vi "PicoScope4000aExampleStreaming.vi"(1 "stop":bool, 5 "Open Using Serial Number":bool, 7 "Serial Number":string) -> ()   [LabVIEW 2010]
doc: "This example demonstrates how to use the PicoScope Labview library to stream data from a PicoScope 5000 Series Device"
uses:
  PicoScope4000aLib/PicoScope4000aAnalogChannelSettings.ctl
  shared/Buffer and Transfer Settings.ctl
panel:
  in  "Write to TDMS":bool
  out "Unit Info":T1
  in  "Trigger Settings":T2={"Trigger Enabled"=FALSE, "Trigger Source"=enum."Channel A", "Trigger Threshold (Volts/Probe units)"=0.0, "Trigger Direction"=2, "Trigger Delay (samples)"=0, "Auto Trigger Time (ms)"=1000} {"Trigger Direction" items=["Rising"=2, "Falling"=3]}
  out "Analog Channels":cluster{i32, dbl, "Data (Volts)":dbl[]}[](graph)
  in  "Channel B Settings":T3={"Enabled"=TRUE, "Coupling"=1, "Range"=6, "Analogue Offset"=0.0, "Bandwidth Limit"=0} {"Bandwidth Limit" items=["Full", "20kHz", "100kHz", "1MHz"]; "Range" items=["10 mV", "20 mV", "50 mV", "100 mV", "200 mV", "500 mV", "1 V", "2 V", "5 V", "10 V", "20 V", "50 V ", "100 V"]; "Coupling" items=["AC", "DC"]}
  in  "Channel A Settings":T3={"Enabled"=TRUE, "Coupling"=1, "Range"=6, "Analogue Offset"=0.0, "Bandwidth Limit"=0} {"Bandwidth Limit" items=["Full", "20kHz", "100kHz", "1MHz"]; "Range" items=["10 mV", "20 mV", "50 mV", "100 mV", "200 mV", "500 mV", "1 V", "2 V", "5 V", "10 V", "20 V", "50 V ", "100 V"]; "Coupling" items=["AC", "DC"]}
  out "Raw Sample Interval (sec)":dbl format="%#.5p"
  out "Max ADC value":i16
  out "Chunk time(ms)":u32
  out "Elapsed time":dbl
  in  "Data file":path=path "PicoScope4000aExampleStreaming Data"
  out "Queue depth":i32(graph)
  out "queue depth":i32
  in  "Buffer and Transfer Settings":T4={"startIndex"=0, "Samples"=1000000, "Down Sample Ratio"=1, "Down-Sample Mode"=0} {"Down-Sample Mode" items=["RAW none"=2147483648, "None"=0, "Aggregate"=1, "Decimate"=2, "Average"=4]; "Down Sample Ratio" step=1; "Samples" format="%_6p"}
  out "USB Powered":bool
  out "USB 3.0 device on non-USB 3.0 Port":bool=TRUE
  out "TriggeredAt (In Buffer)":u32 format="%#.6p"
  out "TriggeredAt (Total samples)":u32 format="%#.6p"
  in  "Acquisition Settings":T5={"Auto Stop"=FALSE, "Desired Sample Interval"=100, "Pre-trigger Samples"=0, "Post-trigger Samples"=1000000, "Down-Sample Ratio"=1, "Down-Sample Mode"=0, "Time Units"=2} {"Time Units" items=["Nanoseconds (ns)"=2, "Microseconds (us)"=3, "Milliseconds (ms)"=4, "Seconds (s)"=5]; "Down-Sample Mode" items=["None"=0, "Aggregate"=1, "Decimate"=2, "Average"=4]; "Post-trigger Samples" format="%#.6p"; "Pre-trigger Samples" format="%#_6p"}
  out "Triggered":bool
  out "DownSample Interval (sec)":dbl format="%#.5p"
  out "Total Samples":u32 format="%#.6p"
  out "Auto Stopped":bool
  out "Number of Samples per Capture":u32 format="%#.6p"
  in  "Resolution":u32(ring)=1 items=["8-bit", "12-bit", "14-bit", "15-bit (max. 2 ch.)", "16-bit (max. 1 ch.)"]
  in  "Apply  Settings":bool
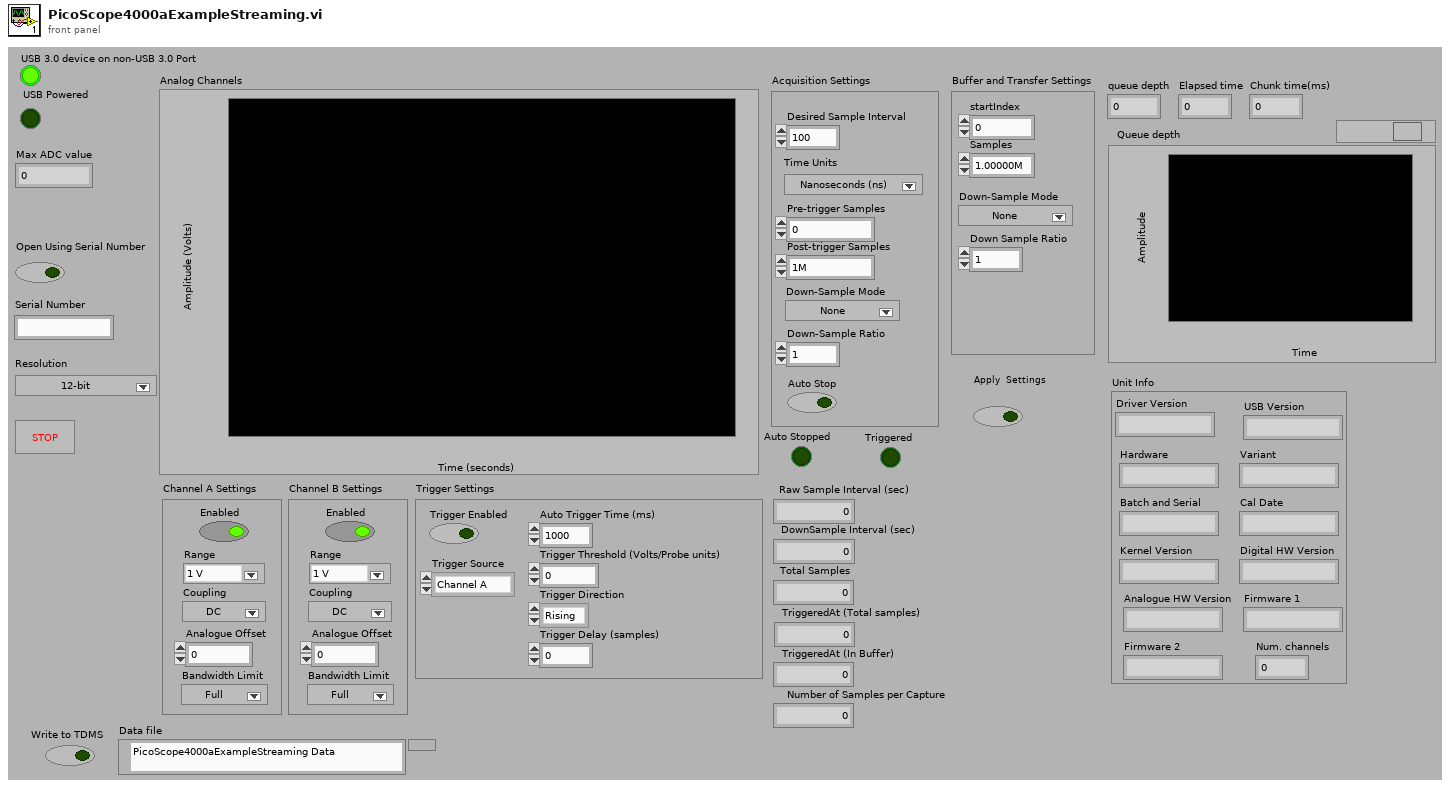
[diagram p1: front panel]
types:
  T1 = cluster{"Driver Version":string, "USB Version":string, "Hardware":string, "Variant":string, "Batch and Serial":string, "Cal Date":string, "Kernel Version":string, "Digital HW Version":string, "Analogue HW Version":string, "Firmware 1":string, "Firmware 2":string, "Num. channels":i16}
  T2 = cluster{"Trigger Enabled":bool, "Trigger Source":enum16{"Channel A", "Channel B", "Channel C", "Channel D", "Channel E", "Channel F", "Channel G", "Channel H"}, "Trigger Threshold (Volts/Probe units)":dbl, "Trigger Direction":u16, "Trigger Delay (samples)":u32, "Auto Trigger Time (ms)":i16}
  T3 = typedef "PicoScope4000aAnalogChannelSettings.ctl" = cluster{"Enabled":bool, "Coupling":i16, "Range":u32, "Analogue Offset":sgl, "Bandwidth Limit":u32}
  T4 = typedef "Buffer and Transfer Settings.ctl" = cluster{"startIndex":u64, "Samples":u64, "Down Sample Ratio":u64, "Down-Sample Mode":u32}
  T5 = cluster{"Auto Stop":bool, "Desired Sample Interval":u32, "Pre-trigger Samples":u32, "Post-trigger Samples":u32, "Down-Sample Ratio":u32, "Down-Sample Mode":i32, "Time Units":u32}
  T6 = enum16{"open", "open or create", "create or replace", "create", "open (read-only)"}
  T7 = cluster{"Channel A Buffer":i16[], "Channel B Buffer":i16[], "Channel C Buffer":i16[], "Channel D Buffer":i16[], "Channel E Buffer":i16[], "Channel F Buffer":i16[], "Channel G Buffer":i16[], "Channel H Buffer":i16[], "Port 0":i16[], "Port 1":i16[]}
  T8 = cluster{i32, "DownSample Interval (sec)":dbl, "Data":dbl[]}
  T9 = cluster{i32, "DownSample Interval (sec)":dbl, "Data":dbl[]}[]
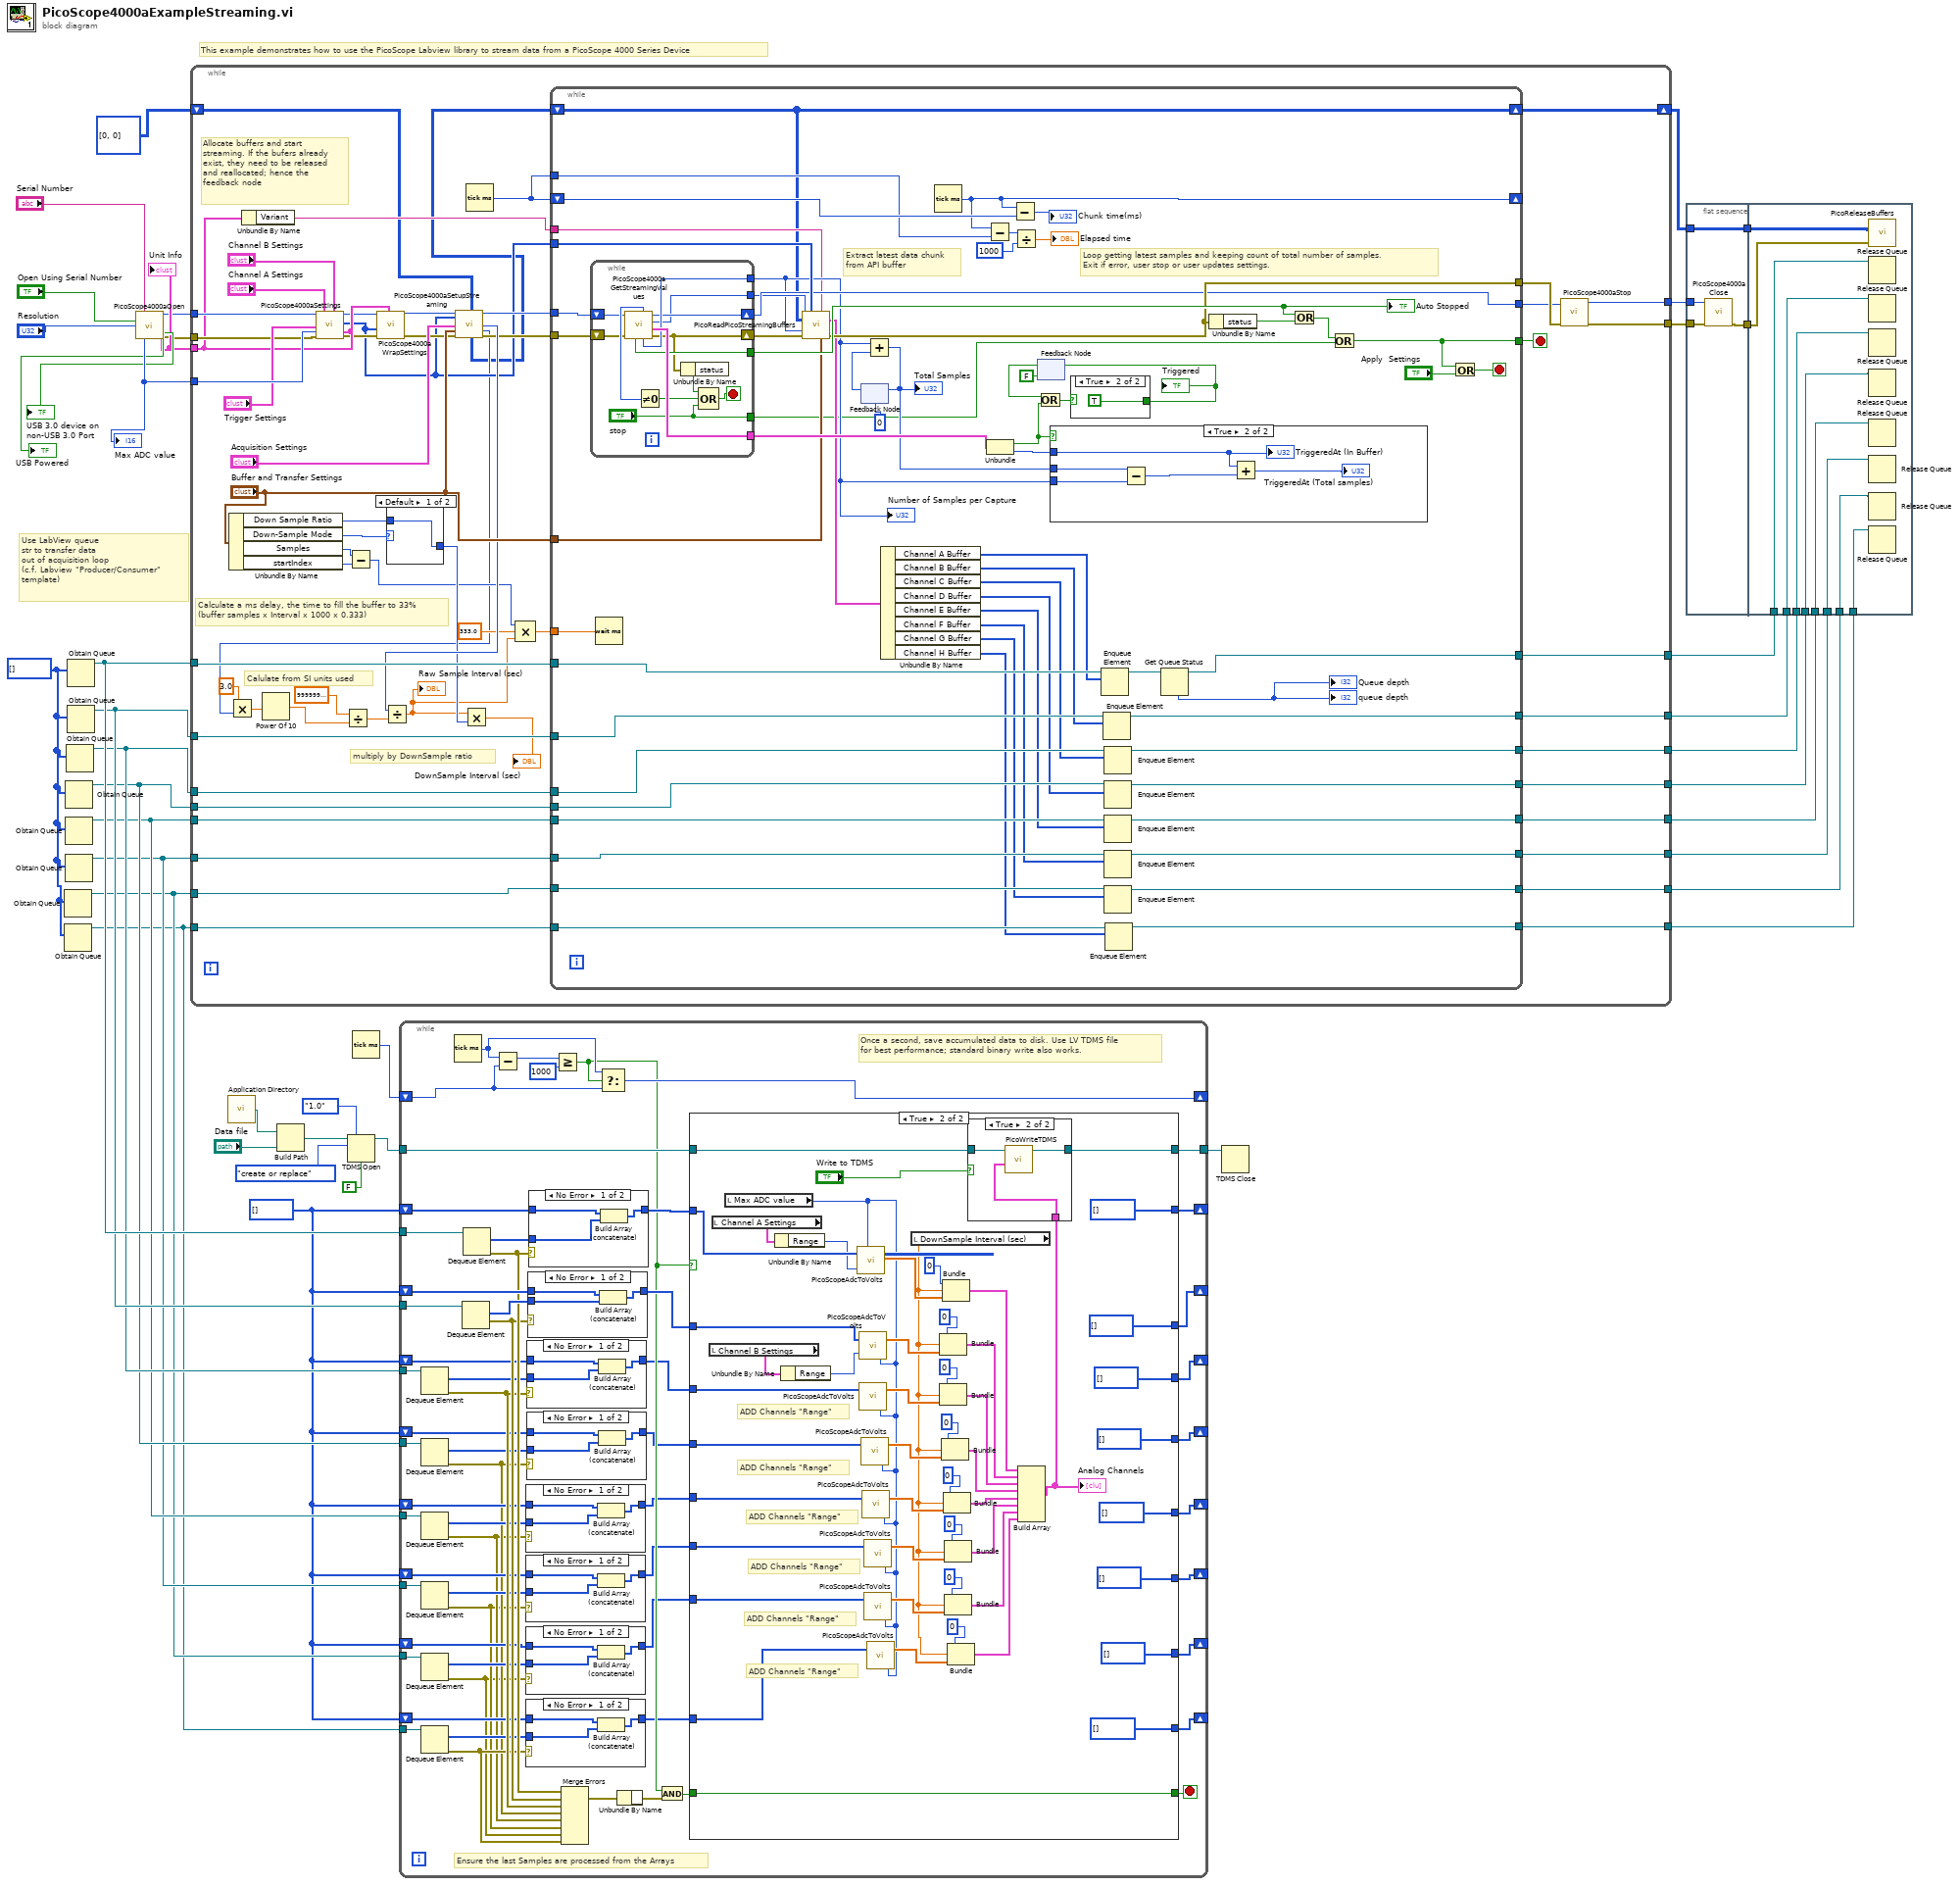
[diagram p0: block diagram]
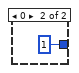
[diagram p12: hidden frame]
diagram:
  w8 = i16[] [] ("History Data")
  w21 = i16[] [] ("History Data")
  # "Use LabView queue\nstr to transfer data\nout of acquisition loop\n(c.f. Labview \"Producer/Consumer\"\ntemplate)"
  # "This example demonstrates how to use the PicoScope Labview library to stream data from a PicoScope 4000 Series Device"
  n1 = Obtain Queue(element data type=w21) -> (queue out=w10:refnum<queue>)  [unwired: 4 in, 2 out]
  n2 = Obtain Queue(element data type=w21) -> (queue out=w9:refnum<queue>)  [unwired: 4 in, 2 out]
  n3 = Obtain Queue(element data type=w21) -> (queue out=w13:refnum<queue>)  [unwired: 4 in, 2 out]
  n4 = Obtain Queue(element data type=w21) -> (queue out=w12:refnum<queue>)  [unwired: 4 in, 2 out]
  n5 = Obtain Queue(element data type=w21) -> (queue out=w11:refnum<queue>)  [unwired: 4 in, 2 out]
  n6 = Obtain Queue(element data type=w21) -> (queue out=w14:refnum<queue>)  [unwired: 4 in, 2 out]
  n7 = Obtain Queue(element data type=w21) -> (queue out=w38:refnum<queue>)  [unwired: 4 in, 2 out]
  n8 = Obtain Queue(element data type=w21) -> (queue out=w26:refnum<queue>)  [unwired: 4 in, 2 out]
  n9 = call "PicoScope4000aOpen.vi"("Serial Number"="Serial Number", "Use Serial Number"="Open Using Serial Number", "Resolution"="Resolution") -> ("handle"=w6:i16, "Unit Info"=w22:T1, "Max ADC value"=w39:i16, "USB powered"=→"USB 3.0 device on non-USB 3.0 Port":bool, "USB 3.0 on non-USB 3.0 port"=→"USB Powered":bool, "error out"=w5:errorcluster)  [unwired: 5 in, 2 out]
  "Max ADC value" <- w39
  "Unit Info" <- w22
  n10 = while {
    tunnel: [w87] -> w37
    tunnel: w22 -> [w54]
    tunnel: w39 -> [w100]
    tunnel: [w95] -> w36
    tunnel: w38 -> [w94]
    tunnel: [w93] -> w27
    tunnel: w26 -> [w92]
    tunnel: w14 -> [w74]
    tunnel: w13 -> [w73]
    tunnel: w12 -> [w72]
    tunnel: w11 -> [w71]
    tunnel: w10 -> [w70]
    tunnel: w9 -> [w69]
    tunnel: [w68] -> w20
    tunnel: [w67] -> w19
    tunnel: [w66] -> w18
    tunnel: [w65] -> w17
    tunnel: [w64] -> w16
    tunnel: [w63] -> w15
    tunnel: [w58] -> w7
    tunnel: w6 -> [w56]
    tunnel: w5 -> [w55]
    shift-right: [w43] -> w3
    shift-left: u64[][] [[0], [0]] ("Pointer array") -> [w45]
    stop <- w101 stop-if-true
    # "Calculate a ms delay, the time to fill the buffer to 33%\n(buffer samples x Interval x 1000 x 0.333)"
    # "multiply by DownSample ratio"
    # "Calulate from SI units used"
    # "Allocate buffers and start\nstreaming. If the bufers already\nexist, they need to be released\nand reallocated; hence the\nfeedback node"
    n11 = Unbundle By Name("Buffer and Transfer Settings") -> ("Down Sample Ratio"=w98:u64, "Down-Sample Mode"=w99:u32, "Samples"=w77:u64, "startIndex"=w76:u64)
    n12 = Unbundle By Name(w54) -> ("Variant"=w59:string)
    n13 = call "PicoScope4000aSettings.vi"("handle in"=w56, "Trigger Settings"="Trigger Settings", "Max ADC value"=w100, "error in"=w55, "Channel A Settings"="Channel A Settings", "Channel B Settings"="Channel B Settings", "Unit Info"=w54) -> ("handle out"=w52:i16, "Enabled array"=w47:i16[], "error out"=w53:errorcluster)  [unwired: 10 in]
    n14 = Subtract(x=w77, y=w76) -> (x-y=w61:u64)
    n15 = call "PicoScope4000aWrapSettings.vi"("Unit Info"=w54, "error in (no error)"=w53, "Enabled array"=w47, "Handle In"=w52) -> ("error out"=w49:errorcluster, "Handle Out"=w48:i16)  [unwired: 6 in]
    n16 = case shown="Default" w99 {
      tunnel: [w102 u32 1 ("Down-Sample Ratio")] -> w79
      tunnel: w98 -> [w102 _]
      frame Default {
      }
      frame 0 {
      }
    }
    n17 = call "PicoScope4000aSetupStreaming.vi"("handle in"=w48, "enabled array"=w47, "Acquisition Settings"="Acquisition Settings", "Buffer and Transfer Settings"="Buffer and Transfer Settings", "error in"=w49, "Pointers In"=w45) -> ("Pointer array"=w44:u64[][], "handle out"=w51:i16, "Sample Interval"=w80:u32, "sampleIntervalTimeUnits"=w46:u32, "error out"=w50:errorcluster)  [unwired: 9 in]
    n18 = Multiply(x=3.0, y=w46) -> (x*y=w85:dbl)
    n19 = Power Of 10(x=w85) -> (10^x=w84:dbl)
    n20 = Divide(x=sgl 1000000000000000.0 ("y"), y=w84) -> (x/y=w81:dbl)
    n21 = Divide(x=w80, y=w81) -> (x/y=w60:dbl)
    "Raw Sample Interval (sec)" <- w60
    n22 = Multiply(x=w60, y=w79) -> (x*y=→"DownSample Interval (sec)":dbl)
    n23 = Tick Count (ms)() -> (millisecond timer value=w86:u32)
    n24 = Compound Arithmetic op=MULTIPLY(w61, 333.0 ("value"), w60) -> (w78:dbl)
    n25 = while {
      tunnel: [w133] -> w88
      tunnel: [w165] -> w101
      tunnel: w51 -> [w150]
      tunnel: w50 -> [w149]
      tunnel: [w146] -> w89
      tunnel: "Buffer and Transfer Settings" -> [w148]
      tunnel: w47 -> [w145]
      tunnel: [w143] -> w95
      tunnel: w94 -> [w141]
      shift-right: [w135] -> _
      shift-left: w86 -> [w136]
      tunnel: w59 -> [w129]
      tunnel: [w124] -> w93
      tunnel: w92 -> [w128]
      tunnel: w86 -> [w125]
      tunnel: w78 -> [w105]
      tunnel: w74 -> [w123]
      tunnel: w73 -> [w122]
      tunnel: w72 -> [w121]
      tunnel: w71 -> [w120]
      tunnel: w70 -> [w119]
      tunnel: w69 -> [w118]
      tunnel: [w117] -> w68
      tunnel: [w116] -> w67
      tunnel: [w115] -> w66
      tunnel: [w114] -> w65
      tunnel: [w113] -> w64
      tunnel: [w112] -> w63
      shift-right: [w104] -> w43
      shift-left: w44 -> [w104]
      stop <- w164 stop-if-true
      # "Loop getting latest samples and keeping count of total number of samples. \nExit if error, user stop or user updates settings."
      # "Extract latest data chunk\nfrom API buffer"
      n26 = while {
        tunnel: [w179] -> w163
        tunnel: [w178] -> w160
        tunnel: [w167] -> w131
        tunnel: [w177] -> w130
        shift-right: [w168] -> w133
        shift-left: w150 -> [w171]
        shift-right: [w169] -> w147
        shift-left: w149 -> [w170]
        tunnel: ["stop"] -> w126
        stop <- w173 stop-if-true
        n27 = call "PicoScope4000aGetStreamingValues.vi"("error in"=w170, "handle in"=w171) -> ("error out"=w169:errorcluster, "Trigger"=w179:cluster{bool, "triggeredAt (Total samples)":u32}, "Start Index in Driver Buffer"=w167:u32, "handle out"=w168:i16, "Number of Samples"=w177:u32, "ready"=w176:i16, "Auto Stopped"=w178:bool)  [unwired: 3 in]
        n28 = Not Equal To 0?(x=w176) -> (x != 0?=w174:bool)
        n29 = Unbundle By Name(w169) -> ("status"=w175:bool)
        n30 = Compound Arithmetic op=OR(w175, w174, "stop") -> (w173:bool)
      }
      "Number of Samples per Capture" <- w130
      "Auto Stopped" <- w160
      n31 = Wait (ms)(milliseconds to wait=w105) -> ()  [unwired: 1 out]
      n32 = call "PicoReadPicoStreamingBuffers.vi"("enabled array"=w145, "Buffer and Transfer Settings"=w148, "Variant"=w129, "Pointer array"=w104, "Offset Index"=w131, "Number of Samples"=w130, "error in (no error)"=w147) -> ("Buffers (Max or non-aggregated)"=w140:T7, "error out"=w146:errorcluster)  [unwired: 6 in, 1 out]
      n33 = feedback #1(u32 0) -> (w156:u32)
      n34 = Add(x=w130, y=w156) -> (x+y=w154:u32)
      "Total Samples" <- w154
      n35 = feedback-in #1(w154) -> ()
      n36 = Unbundle By Name(w140) -> ("Channel A Buffer"=w132:i16[], "Channel B Buffer"=w127:i16[], "Channel C Buffer"=w111:i16[], "Channel D Buffer"=w110:i16[], "Channel E Buffer"=w109:i16[], "Channel F Buffer"=w108:i16[], "Channel G Buffer"=w107:i16[], "Channel H Buffer"=w106:i16[])
      n37 = Tick Count (ms)() -> (millisecond timer value=w135:u32)
      n38 = Subtract(x=w135, y=w125) -> (x-y=w139:u32)
      n39 = Unbundle(w163) -> (w152:bool, "triggeredAt (Total samples)"=w151:u32)
      n40 = Subtract(x=w135, y=w136) -> (x-y=→"Chunk time(ms)":u32)
      n41 = Divide(x=w139, y=u32 1000) -> (x/y=→"Elapsed time":dbl)
      n42 = feedback #2(FALSE) -> (w158:bool)
      n43 = Or(x=w158, y=w152) -> (x .or. y?=w155:bool)
      n44 = case shown="True" w152 {
        tunnel: w130 -> [_ w180]
        tunnel: w154 -> [_ w184]
        tunnel: w151 -> [_ w182]
        frame False {
        }
        frame True {
          n45 = Subtract(x=w184, y=w180) -> (x-y=w183:u32)
          n46 = Add(x=w182, y=w183) -> (x+y=→"TriggeredAt (Total samples)":u32)
          "TriggeredAt (In Buffer)" <- w182
        }
      }
      n47 = case shown="True" w155 {
        selector: w155 -> [w185 _]
        tunnel: [w185 TRUE] -> w153
        frame False {
        }
        frame True {
        }
      }
      "Triggered" <- w153
      n48 = feedback-in #2(w153) -> ()
      n49 = Enqueue Element(queue=w141, element=w132) -> (queue out=w142:refnum<queue>)  [unwired: 2 in, 2 out]
      n50 = Enqueue Element(queue=w128, element=w127) -> (queue out=w124:refnum<queue>)  [unwired: 2 in, 2 out]
      n51 = Enqueue Element(queue=w123, element=w111) -> (queue out=w117:refnum<queue>)  [unwired: 2 in, 2 out]
      n52 = Enqueue Element(queue=w122, element=w110) -> (queue out=w116:refnum<queue>)  [unwired: 2 in, 2 out]
      n53 = Enqueue Element(queue=w121, element=w109) -> (queue out=w115:refnum<queue>)  [unwired: 2 in, 2 out]
      n54 = Enqueue Element(queue=w120, element=w108) -> (queue out=w114:refnum<queue>)  [unwired: 2 in, 2 out]
      n55 = Enqueue Element(queue=w119, element=w107) -> (queue out=w113:refnum<queue>)  [unwired: 2 in, 2 out]
      n56 = Enqueue Element(queue=w118, element=w106) -> (queue out=w112:refnum<queue>)  [unwired: 2 in, 2 out]
      n57 = Get Queue Status(queue=w142) -> (queue out=w143:refnum<queue>, # elements in queue=→"queue depth" →"Queue depth":i32)  [unwired: 2 in, 6 out]
      n58 = Unbundle By Name(w146) -> ("status"=w162:bool)
      n59 = Or(x=w160, y=w162) -> (x .or. y?=w161:bool)
      n60 = Or(x=w161, y=w126) -> (x .or. y?=w165:bool)
      n61 = Or(x=w165, y="Apply  Settings") -> (x .or. y?=w164:bool)
    }
    n62 = call "PicoScope4000aStop.vi"("error in (no error)"=w89, "handle in"=w88) -> ("error out"=w58:errorcluster, "handle out"=w87:i16)  [unwired: 8 in]
  }
  n63 = call <vilib>:"Application Directory.vi"() -> ("Application Directory"=w23:path)
  n64 = Build Path(base path=w23, name or relative path="Data file") -> (appended path=w24:path)
  n65 = TDMS Open(6:FALSE ("disable buffering? (T)"), 7:enum16{"1.0", "2.0"}."1.0" ("file format version (2.0)"), 10:T6."create or replace" ("operation (0:open)"), 11:w24) -> (3:w31:refnum<k34>)  [unwired: 2 in, 1 out]
  n66 = Tick Count (ms)() -> (millisecond timer value=w33:u32)
  n67 = while {
    tunnel: w38 -> [w245]
    shift-right: [w237] -> _
    shift-left: w8 -> [w244]
    shift-right: [w239] -> _
    shift-left: w33 -> [w240]
    tunnel: w31 -> [w236]
    tunnel: [w235] -> w30
    tunnel: w26 -> [w233]
    shift-right: [w230] -> _
    shift-left: w8 -> [w232]
    tunnel: w14 -> [w223]
    tunnel: w13 -> [w222]
    tunnel: w12 -> [w221]
    tunnel: w11 -> [w220]
    tunnel: w10 -> [w219]
    tunnel: w9 -> [w218]
    shift-right: [w193] -> _
    shift-left: w8 -> [w216]
    shift-right: [w194] -> _
    shift-left: w8 -> [w207]
    shift-right: [w195] -> _
    shift-left: w8 -> [w206]
    shift-right: [w196] -> _
    shift-left: w8 -> [w203]
    shift-right: [w197] -> _
    shift-left: w8 -> [w201]
    shift-right: [w198] -> _
    shift-left: w8 -> [w208]
    stop <- w227 stop-if-true
    # "Ensure the last Samples are processed from the Arrays"
    # "Once a second, save accumulated data to disk. Use LV TDMS file\nfor best performance; standard binary write also works."
    n68 = Dequeue Element(queue=w223) -> (element=w215:i16[], error out=w217:errorcluster)  [unwired: 2 in, 2 out]
    n69 = Dequeue Element(queue=w222) -> (element=w205:i16[], error out=w191:errorcluster)  [unwired: 2 in, 2 out]
    n70 = Dequeue Element(queue=w221) -> (element=w204:i16[], error out=w190:errorcluster)  [unwired: 2 in, 2 out]
    n71 = Dequeue Element(queue=w220) -> (element=w202:i16[], error out=w189:errorcluster)  [unwired: 2 in, 2 out]
    n72 = Dequeue Element(queue=w219) -> (element=w200:i16[], error out=w188:errorcluster)  [unwired: 2 in, 2 out]
    n73 = Dequeue Element(queue=w218) -> (element=w199:i16[], error out=w192:errorcluster)  [unwired: 2 in, 2 out]
    n74 = Tick Count (ms)() -> (millisecond timer value=w241:u32)
    n75 = Dequeue Element(queue=w233) -> (element=w234:i16[], error out=w228:errorcluster)  [unwired: 2 in, 2 out]
    n76 = Dequeue Element(queue=w245) -> (element=w246:i16[], error out=w229:errorcluster)  [unwired: 2 in, 2 out]
    n77 = Subtract(x=w241, y=w240) -> (x-y=w243:u32)
    n78 = case shown="No Error" w190 {
      tunnel: w206 -> [w261 w262]
      tunnel: [w260 w262] -> w212
      tunnel: w204 -> [w259 _]
      frame No Error {
        n79 = Build Array (concatenate)(w261, w259) -> (w260:i16[])
      }
      frame Error {
      }
    }
    n80 = case shown="No Error" w189 {
      tunnel: w203 -> [w257 w258]
      tunnel: [w256 w258] -> w211
      tunnel: w202 -> [w255 _]
      frame No Error {
        n81 = Build Array (concatenate)(w257, w255) -> (w256:i16[])
      }
      frame Error {
      }
    }
    n82 = case shown="No Error" w188 {
      tunnel: w201 -> [w253 w254]
      tunnel: [w252 w254] -> w210
      tunnel: w200 -> [w251 _]
      frame No Error {
        n83 = Build Array (concatenate)(w253, w251) -> (w252:i16[])
      }
      frame Error {
      }
    }
    n84 = case shown="No Error" w192 {
      tunnel: w208 -> [w249 w250]
      tunnel: [w248 w250] -> w209
      tunnel: w199 -> [w247 _]
      frame No Error {
        n85 = Build Array (concatenate)(w249, w247) -> (w248:i16[])
      }
      frame Error {
      }
    }
    n86 = case shown="No Error" w217 {
      tunnel: w216 -> [w269 w270]
      tunnel: [w268 w270] -> w214
      tunnel: w215 -> [w267 _]
      frame No Error {
        n87 = Build Array (concatenate)(w269, w267) -> (w268:i16[])
      }
      frame Error {
      }
    }
    n88 = case shown="No Error" w191 {
      tunnel: w207 -> [w265 w266]
      tunnel: [w264 w266] -> w213
      tunnel: w205 -> [w263 _]
      frame No Error {
        n89 = Build Array (concatenate)(w265, w263) -> (w264:i16[])
      }
      frame Error {
      }
    }
    n90 = case shown="No Error" w228 {
      tunnel: w232 -> [w273 w274]
      tunnel: [w272 w274] -> w231
      tunnel: w234 -> [w271 _]
      frame No Error {
        n91 = Build Array (concatenate)(w273, w271) -> (w272:i16[])
      }
      frame Error {
      }
    }
    n92 = case shown="No Error" w229 {
      tunnel: w244 -> [w342 w343]
      tunnel: [w341 w343] -> w238
      tunnel: w246 -> [w340 _]
      frame No Error {
        n93 = Build Array (concatenate)(w342, w340) -> (w341:i16[])
      }
      frame Error {
      }
    }
    n94 = Greater Or Equal?(x=w243, y=u32 1000) -> (x >= y?=w225:bool)
    n95 = Merge Errors(w229, w228, w217, w191, w190, w189, w188, w192) -> (w226:errorcluster)
    n96 = Select(t=w241, s=w225, f=w240) -> (s? t:f=w239:u32)
    n97 = And(x=w225) -> (y=w187:errorcluster, x .and. y?=w224:bool)
    n98 = Unbundle By Name(w226, w187) -> ()
    n99 = case shown="True" w225 {
      tunnel: w238 -> [w284 w332]
      tunnel: [w284 i16[] [] ("History Data")] -> w237
      tunnel: w236 -> [w283 w334]
      tunnel: [w283 w333] -> w235
      tunnel: w231 -> [w282 w322]
      tunnel: [w282 i16[] [] ("History Data")] -> w230
      tunnel: [w281 w319] -> w227
      tunnel: w224 -> [w281 w319]
      tunnel: w214 -> [w280 w314]
      tunnel: w213 -> [w279 w297]
      tunnel: w212 -> [w278 w296]
      tunnel: w211 -> [w277 w295]
      tunnel: w210 -> [w276 w294]
      tunnel: w209 -> [w275 w293]
      tunnel: [w275 i16[] [] ("History Data")] -> w198
      tunnel: [w276 i16[] [] ("History Data")] -> w197
      tunnel: [w277 i16[] [] ("History Data")] -> w196
      tunnel: [w278 i16[] [] ("History Data")] -> w195
      tunnel: [w279 i16[] [] ("History Data")] -> w194
      tunnel: [w280 i16[] [] ("History Data")] -> w193
      frame False {
      }
      frame True {
        # "ADD Channels \"Range\""
        # "ADD Channels \"Range\""
        # "ADD Channels \"Range\""
        # "ADD Channels \"Range\""
        # "ADD Channels \"Range\""
        # "ADD Channels \"Range\""
        n100 = local read "Channel B Settings"() -> (w320:T3)
        n101 = local read "Channel A Settings"() -> (w321:T3)
        n102 = local read "Max ADC value"() -> (w298:i16)
        n103 = Unbundle By Name(w321) -> ("Range"=w331:u32)
        n104 = Unbundle By Name(w320) -> ("Range"=w323:u32)
        n105 = call "PicoScopeAdcToVolts.vi"("Max_adc"=w298, "Range Index"=w331, "Data"=w332) -> ("Data"=w329:dbl[])
        n106 = call "PicoScopeAdcToVolts.vi"("Max_adc"=w298, "Range Index"=w323, "Data"=w322) -> ("Data"=w327:dbl[])
        n107 = call "PicoScopeAdcToVolts.vi"("Max_adc"=w298, "Data"=w314) -> ("Data"=w318:dbl[])  [unwired: 1 in]
        n108 = call "PicoScopeAdcToVolts.vi"("Max_adc"=w298, "Data"=w297) -> ("Data"=w316:dbl[])  [unwired: 1 in]
        n109 = call "PicoScopeAdcToVolts.vi"("Max_adc"=w298, "Data"=w296) -> ("Data"=w313:dbl[])  [unwired: 1 in]
        n110 = call "PicoScopeAdcToVolts.vi"("Max_adc"=w298, "Data"=w295) -> ("Data"=w311:dbl[])  [unwired: 1 in]
        n111 = call "PicoScopeAdcToVolts.vi"("Max_adc"=w298, "Data"=w294) -> ("Data"=w309:dbl[])  [unwired: 1 in]
        n112 = call "PicoScopeAdcToVolts.vi"("Max_adc"=w298, "Data"=w293) -> ("Data"=w307:dbl[])  [unwired: 1 in]
        n113 = local read "DownSample Interval (sec)"() -> (w305:dbl)
        n114 = Bundle(0, "DownSample Interval (sec)"=w305, "Data"=w327) -> (w324:T8)  [unwired: 1 in]
        n115 = Bundle(0, "DownSample Interval (sec)"=w305, "Data"=w318) -> (w304:T8)  [unwired: 1 in]
        n116 = Bundle(0, "DownSample Interval (sec)"=w305, "Data"=w316) -> (w303:T8)  [unwired: 1 in]
        n117 = Bundle(0, "DownSample Interval (sec)"=w305, "Data"=w329) -> (w325:T8)  [unwired: 1 in]
        n118 = Bundle(0, "DownSample Interval (sec)"=w305, "Data"=w313) -> (w302:T8)  [unwired: 1 in]
        n119 = Bundle(0, "DownSample Interval (sec)"=w305, "Data"=w311) -> (w301:T8)  [unwired: 1 in]
        n120 = Bundle(0, "DownSample Interval (sec)"=w305, "Data"=w309) -> (w300:T8)  [unwired: 1 in]
        n121 = Bundle(0, "DownSample Interval (sec)"=w305, "Data"=w307) -> (w299:T8)  [unwired: 1 in]
        n122 = Build Array(w325, w324, w304, w303, w302, w301, w300, w299) -> (w286:T9)
        "Analog Channels" <- w286
        n123 = case shown="True" "Write to TDMS" {
          tunnel: w334 -> [w336 w339]
          tunnel: [w336 w338] -> w333
          tunnel: w286 -> [_ w337]
          frame False {
          }
          frame True {
            n124 = call "PicoWriteTDMS.vi"("Analog Channels"=w337, "Refnum in"=w339) -> ("Refnum out"=w338:refnum<k34>)  [unwired: 8 in, 1 out]
          }
        }
      }
    }
  }
  n125 = TDMS Close(11:w30) -> ()  [unwired: 1 in, 2 out]
  n126 = flat-sequence {
    tunnel: w37 -> [w347]
    tunnel: w7 -> [w346]
    tunnel: w3 -> [w345]
    tunnel: [w345] -> w2
    tunnel: [w344] -> w1
    tunnel: w36 -> [w357]
    tunnel: w27 -> [w356]
    tunnel: w20 -> [w355]
    tunnel: w19 -> [w354]
    tunnel: w18 -> [w353]
    tunnel: w17 -> [w352]
    tunnel: w16 -> [w351]
    tunnel: w15 -> [w350]
    tunnel: w2 -> [w349]
    tunnel: w1 -> [w348]
    frame #0 {
      n127 = call "PicoScope4000aClose.vi"("error in (no error)"=w346, "handle in"=w347) -> ("error out"=w344:errorcluster)  [unwired: 7 in, 1 out]
    }
    frame #1 {
      n128 = call "PicoReleaseBuffers.vi"("error in (no error)"=w348, "Pointer array"=w349) -> ()  [unwired: 8 in, 2 out]
      n129 = Release Queue(queue=w357) -> ()  [unwired: 2 in, 3 out]
      n130 = Release Queue(queue=w356) -> ()  [unwired: 2 in, 3 out]
      n131 = Release Queue(queue=w355) -> ()  [unwired: 2 in, 3 out]
      n132 = Release Queue(queue=w354) -> ()  [unwired: 2 in, 3 out]
      n133 = Release Queue(queue=w353) -> ()  [unwired: 2 in, 3 out]
      n134 = Release Queue(queue=w352) -> ()  [unwired: 2 in, 3 out]
      n135 = Release Queue(queue=w351) -> ()  [unwired: 2 in, 3 out]
      n136 = Release Queue(queue=w350) -> ()  [unwired: 2 in, 3 out]
    }
  }
